vi "QueryData.vi"(8 "error in (no error)":errorcluster, 10 "Query?":bool, 11 "PW3390 in":refnum<class "PW3390.lvclass">) -> (0 "error out":errorcluster, 3 "PW3390 out":refnum<class "PW3390.lvclass">)   [LabVIEW 2024, in "PW3390 Actor.lvlib" / "PW3390.lvclass"]
uses:
  PW3390.lvclass
  PW3390.lvclass/PW3390.ctl
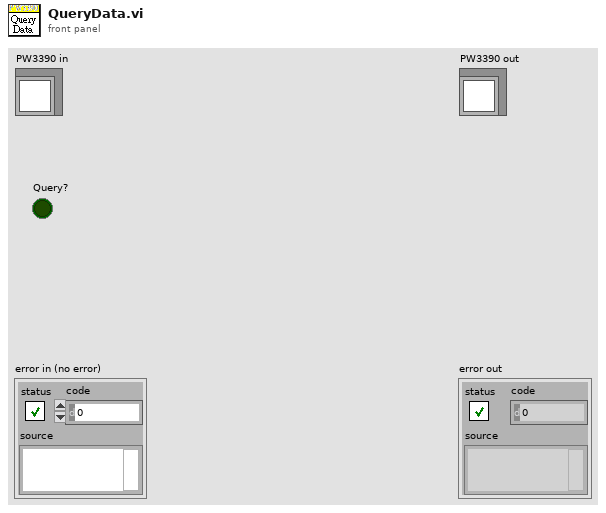
[diagram p1: front panel]
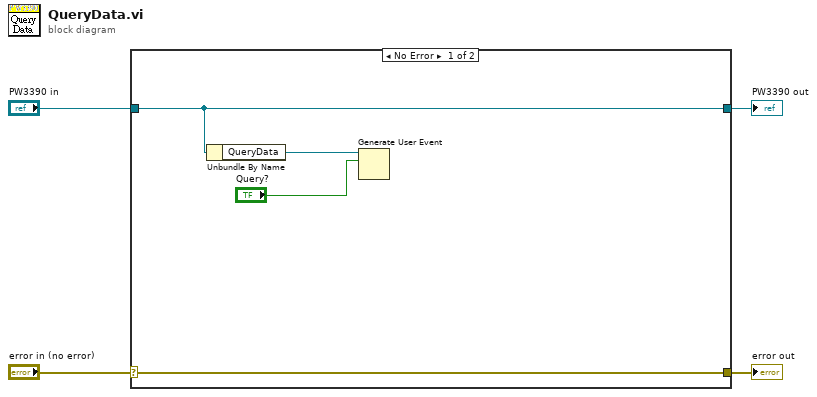
[diagram p0: block diagram]
diagram:
  n1 = case shown="No Error" "error in (no error)" {
    selector: "error in (no error)" -> [w8 w10]
    tunnel: [w8 w10] -> w3
    tunnel: [w7 w9] -> w1
    tunnel: "PW3390 in" -> [w7 w9]
    frame No Error {
      n2 = Unbundle By Name(w7) -> ("QueryData"=w6:refnum<user-event>)
      n3 = Generate User Event(user event=w6, event data cluster="Query?") -> ()  [unwired: 2 in, 2 out]
    }
    frame Error {
    }
  }
  "error out" <- w3
  "PW3390 out" <- w1
